vi "testLeaks.vi"() -> ()   [LabVIEW 2009, in "run.lvlib"]
uses:
  Hal/testing/run.lvlib
  DatabaseHelpers/DbConnection/DeviceDataBase/deviceDataBase.lvclass
panel:
  out "Waveform Chart":dbl(graph)
  in  "stop":bool
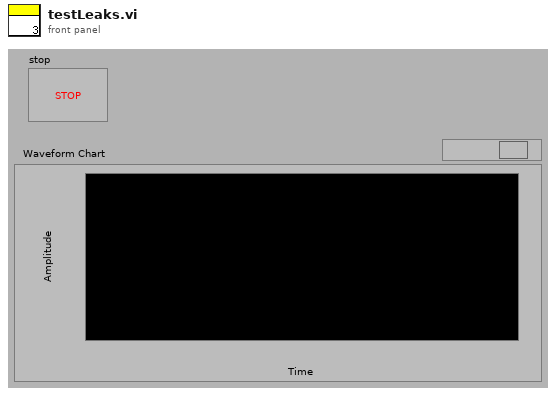
[diagram p1: front panel]
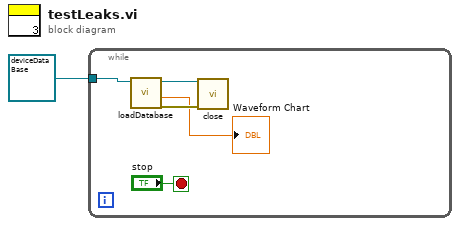
[diagram p0: block diagram]
diagram:
  n1 = while {
    tunnel: refnum<class "deviceDataBase.lvclass"> refnum ("deviceDataBase in") -> [w3]
    stop <- "stop" stop-if-true
    n2 = call "loadDatabase.vi"("deviceDataBase in"=w3) -> ("error out"=w4:errorcluster, "total"=→"Waveform Chart":dbl, "deviceDataBase out"=w5:refnum<class "deviceDataBase.lvclass">)  [unwired: 8 in]
    n3 = call "close.vi"("error in (no error)"=w4, "deviceDataBase in"=w5) -> ()  [unwired: 9 in, 1 out]
  }
